vi "Item_OnCommand.vi"(10 "Command ID":string, 11 "Item Ref":T1) -> ()   [LabVIEW 2020, in "FlexWorker_Provider.lvlib"]
uses:
  <resource>/Framework/Providers/API/ItemRef.ctl
  FlexWorker_Provider.lvlib
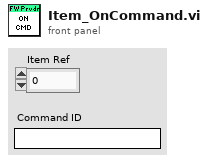
[diagram p1: front panel]
types:
  T1 = typedef "ItemRef.ctl" = u64
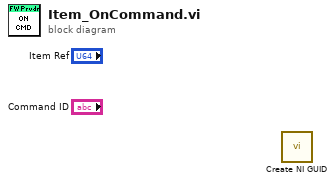
[diagram p0: block diagram]
diagram:
  n1 = call <vilib>:"Create NI GUID.vi"() -> ()  [unwired: 1 out]
